vi "Single Input Attenuation Query.vi"(8 "error in":errorcluster, 10 "Channel":i32(ring) items=["Input Channel 1", "Input Channel 2", "Input Channel 3", "Input Channel 4"], 11 "Instrument Handle In":i32) -> (0 "error out":errorcluster, 2 "Attenuation":dbl, 3 "Instrument Handle Out":i32)   [LabVIEW 8.6, in "ZTScopeM.lvlib"]
doc: "Query the probe attenuation scale factor for the selected channel."
uses:
  ZTScopeM.lvlib
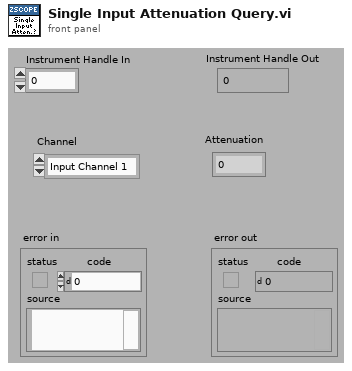
[diagram p1: front panel]
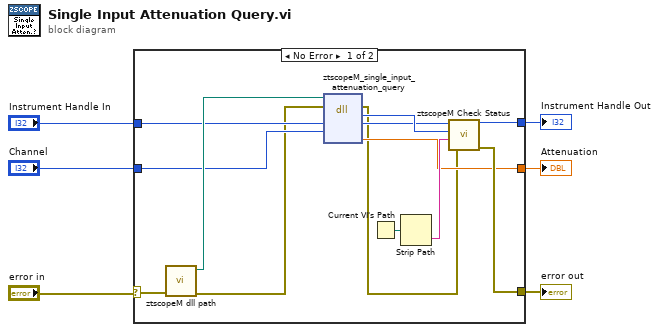
[diagram p0: block diagram]
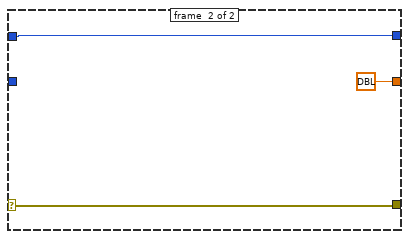
[diagram p2: hidden frame]
diagram:
  n1 = case shown="No Error" "error in" {
    selector: "error in" -> [w12 w22]
    tunnel: [w14 w22] -> w5
    tunnel: [w15 w20] -> w4
    tunnel: [w13 dbl ? ("attenuation")] -> w3
    tunnel: "Instrument Handle In" -> [w10 w20]
    tunnel: "Channel" -> [w9 _]
    frame #0 {
      n2 = call "ztscopeM dll path.vi"("error in (no error)"=w12) -> ("error out"=w8:errorcluster, "<instrument>.dll path"=w11:path)  [unwired: 9 in]
      n3 = dll-call lib="C:/Program Files (x86)/National Instruments/LabVIEW 2013/instr.lib/ztscopem/ztscopeM.dll" fn="ztscopeM_single_input_attenuation_query"(path in=w11, error in=w8, "instrumentHandle"=w10, "channel"=w9) -> (error out=w7:errorcluster, w19:i32, "instrumentHandle"=w18:i32, "attenuation"=w13:dbl)  [unwired: 2 in, 2 out]
      n4 = Current VI's Path() -> (path=w17:path)
      n5 = Strip Path(path=w17) -> (name=w16:string)  [unwired: 1 out]
      n6 = call "ztscopeM Check Status.vi"("error in"=w7, "name of VI"=w16, "status (return code)"=w19, "instrument handle in"=w18) -> ("error out"=w14:errorcluster, "instrument handle out"=w15:i32)  [unwired: 2 out]
    }
    frame #1 {
    }
  }
  "Instrument Handle Out" <- w4
  "error out" <- w5
  "Attenuation" <- w3
